vi "ZLIB Convert File Info__ogtk.vi"(1 "comment":string, 2 "extra field":string, 3 "uncompress file info in":T2 {"external fa" format="%.0x"; "internal fa" format="%.0x"; "crc" format="%.0x"}) -> (0 "file info out":T1 {"file timestamp" format="%<%H:%M:%S\n%d/%m/%Y>T"; "external fa" format="%.0x"; "internal fa" format="%.0x"; "crc" format="%.0x"})   [LabVIEW 2014]
doc: "Convert the file information from the ZIP API format to our LabVIEW format."
uses:
  ZLIB File Info__ogtk.ctl
  ZLIB Uncompress File Info__ogtk.ctl
panel:
  in  "dummy file info":T1 {"file timestamp" format="%<%H:%M:%S\n%d/%m/%Y>T"; "external fa" format="%.0x"; "internal fa" format="%.0x"; "crc" format="%.0x"}
  # "Please visit http://www.OpenG.org to learn about the\nOpen Source LabVIEW software movement.\n\nNOTICE -- YOU MUST LEAVE THIS NOTICE IN PLACE.  PER THE TERMS OF THE LICENSE BELOW, YOU MAY SUBLICENSE THIS SOFTWARE \nIN ANY WAY THAT DOES NOT CONFLICT WITH THIS LICENSE.\n\n### BSD License (http://www.opensource.org/licenses/bsd-license.php) Begin ###\n \nCopyright (C) 2002-2004 Rolf Kalbermatter rolf.kalbermatter@citeng.com\nCopyright (C) 2002 Jim Kring jim@jimkring.com\n\nAll rights reserved.\n\nRedistribution and use in source and binary forms, with or without modification, are permitted provided that the following conditions are met:\n\n    * Redistributions of source code must retain the above copyright notice, this list of conditions and the following disclaimer.\n    * Redistributions in binary form must reproduce the above copyright notice, this list of conditions and the following disclaimer in the \n       documentation and/or other materials provided with the distribution.\n    * Neither the name of SciWare, James Kring, Inc., nor the names of its contributors may be used to endorse or promote products derived \n       from this software without specific prior written permission.\n\nTHIS SOFTWARE IS PROVIDED BY THE COPYRIGHT HOLDERS AND CONTRIBUTORS \"AS IS\" AND ANY EXPRESS OR IMPLIED WARRANTIES, \nINCLUDING, BUT NOT LIMITED TO, THE IMPLIED WARRANTIES OF MERCHANTABILITY AND FITNESS FOR A PARTICULAR PURPOSE ARE \nDISCLAIMED. IN NO EVENT SHALL THE COPYRIGHT OWNER OR CONTRIBUTORS BE LIABLE FOR ANY DIRECT, INDIRECT, INCIDENTAL,\n SPECIAL, EXEMPLARY, OR CONSEQUENTIAL DAMAGES (INCLUDING, BUT NOT LIMITED TO, PROCUREMENT OF SUBSTITUTE GOODS OR \nSERVICES; LOSS OF USE, DATA, OR PROFITS; OR BUSINESS INTERRUPTION) HOWEVER CAUSED AND ON ANY THEORY OF LIABILITY, \nWHETHER IN CONTRACT, STRICT LIABILITY, OR TORT (INCLUDING NEGLIGENCE OR OTHERWISE) ARISING IN ANY WAY OUT OF THE USE \nOF THIS SOFTWARE, EVEN IF ADVISED OF THE POSSIBILITY OF SUCH DAMAGE.\n\n### BSD License End ###"
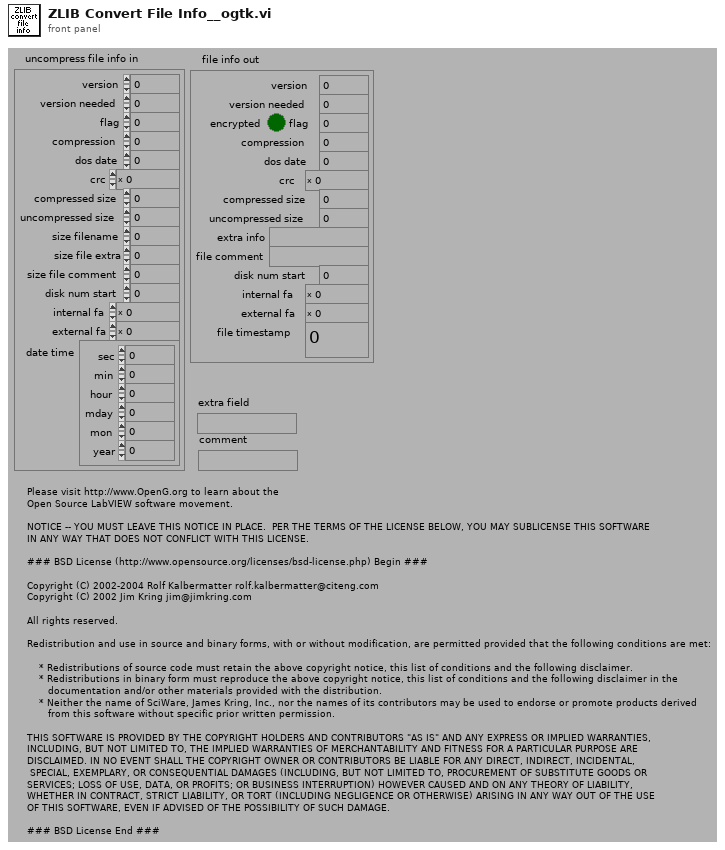
[diagram p1: front panel]
types:
  T1 = typedef "ZLIB File Info__ogtk.ctl" = cluster{"version":u32, "version needed":u32, "encrypted":bool, "flag":u32, "compression":i32, "dos date":u32, "crc":u32, "compressed size":u32, "uncompressed size":u32, "extra info":string, "file comment":string, "disk num start":u32, "internal fa":u32, "external fa":u32, "file timestamp":u32}
  T2 = typedef "ZLIB Uncompress File Info__ogtk.ctl" = cluster{"version":u32, "version needed":u32, "flag":u32, "compression":u32, "dos date":u32, "crc":u32, "compressed size":u32, "uncompressed size":u32, "size filename":u32, "size file extra":u32, "size file comment":u32, "disk num start":u32, "internal fa":u32, "external fa":u32, "date time":cluster{"sec":i32, "min":i32, "hour":i32, "mday":i32, "mon":i32, "year":i32}}
  T3 = cluster{"second":i32, "minute":i32, "hour":i32, "day of month":i32, "month":i32, "year":i32, "day of week":i32, "day of year":i32, "is DST":i32}
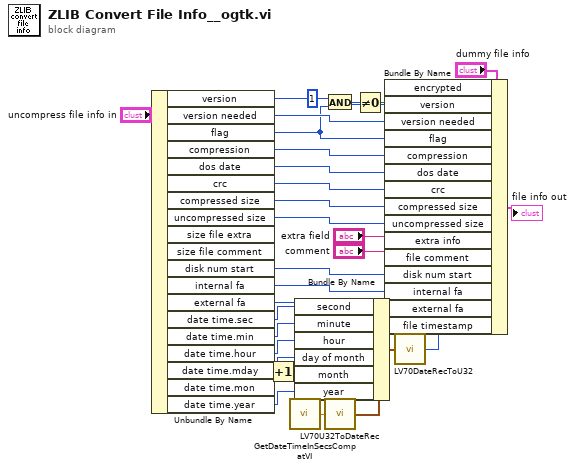
[diagram p0: block diagram]
diagram:
  n1 = Unbundle By Name("uncompress file info in") -> ("version"=w20:u32, "version needed"=w19:u32, "flag"=w18:u32, "compression"=w17:u32, "dos date"=w16:u32, "crc"=w15:u32, "compressed size"=w14:u32, "uncompressed size"=w13:u32, "disk num start"=w12:u32, "internal fa"=w11:u32, "external fa"=w10:u32, "date time.sec"=w23:i32, "date time.min"=w24:i32, "date time.hour"=w25:i32, "date time.mday"=w26:i32, "date time.mon"=w27:i32, "date time.year"=w28:i32)  [unwired: 2 out]
  n2 = Increment(x=w27) -> (x+1=w7:i32)
  n3 = call <vilib>:"GetDateTimeInSecsCompatVI.vi"() -> ("double precision float"=w1:dbl)  [unwired: 1 in]
  n4 = And(x=u32 1, y=w18) -> (x .and. y?=w3:u32)
  n5 = call <vilib>:"LV70U32ToDateRec.vi"("Time"=w1) -> ("date time rec"=w29:T3)
  n6 = Bundle By Name(cluster=w29, "second"=w23, "minute"=w24, "hour"=w25, "day of month"=w26, "month"=w7, "year"=w28) -> (w22:T3)
  n7 = Not Equal To 0?(x=w3) -> (x != 0?=w2:bool)
  n8 = call <vilib>:"LV70DateRecToU32.vi"("date time rec"=w22) -> ("Time"=w9:u32)
  n9 = Bundle By Name(cluster="dummy file info", "encrypted"=w2, "version"=w20, "version needed"=w19, "flag"=w18, "compression"=w17, "dos date"=w16, "crc"=w15, "compressed size"=w14, "uncompressed size"=w13, "extra info"="extra field", "file comment"="comment", "disk num start"=w12, "internal fa"=w11, "external fa"=w10, "file timestamp"=w9) -> (→"file info out":T1)
